vi "draw horizon y.vi"(11 "angle in degrees in":dbl) -> (3 "x-y graph":cluster{"t":dbl[], "t":dbl[]})   [LabVIEW 2016]
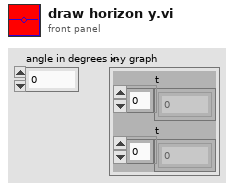
[diagram p1: front panel]
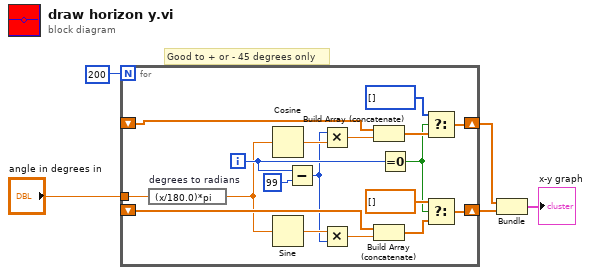
[diagram p0: block diagram]
diagram:
  # "Good to + or - 45 degrees only"
  n1 = for {
    N: 200 -> [_]
    shift-right: [w20] -> w1
    shift-left: _ -> [w23]
    shift-right: [w18] -> w2
    shift-left: _ -> [w21]
    tunnel: "angle in degrees in" -> [w13]
    i -> [w14]
    n2 = expression code="(x/180.0)*pi" "degrees to radians"(w13) -> (w11:dbl)
    n3 = Cosine(x=w11) -> (cos(x)=w12:dbl)
    n4 = Sine(x=w11) -> (sin(x)=w10:dbl)
    n5 = Subtract(x=w14, y=99) -> (x-y=w9:i32)
    n6 = Multiply(x=w9, y=w12) -> (x*y=w7:dbl)
    n7 = Multiply(x=w10, y=w9) -> (x*y=w6:dbl)
    n8 = Build Array (concatenate)(w23, w7) -> (w22:dbl[])
    n9 = Build Array (concatenate)(w21, w6) -> (w8:dbl[])
    n10 = Equal To 0?(x=w14) -> (x = 0?=w16:bool)
    n11 = Select(t=i32[] [], s=w16, f=w22) -> (s? t:f=w20:dbl[])
    n12 = Select(t=dbl[] [], s=w16, f=w8) -> (s? t:f=w18:dbl[])
  }
  n13 = Bundle("t"=w1, "t"=w2) -> (→"x-y graph":cluster{"t":dbl[], "t":dbl[]})  [unwired: 1 in]
